vi "Check if config file is valid.vi"(8 "error in (no error)":errorcluster, 10 "Root node":string, 11 "DOM":refnum<k20>) -> (0 "error out":errorcluster)   [LabVIEW 2011, in "COSYLib.lvlib" / "CoSy Config File.lvclass"]
doc: "Checks if a loaded config file appears to be valid (i.e., includes a version number and header information).\nIf the file is invalid, \"error out\" is set to -2628."
uses:
  CoSy Config File.lvclass
  <vilib>/xml/Close Reference(Node).vi
  <vilib>/xml/NI_XML.lvlib
  C:/Program Files (x86)/National Instruments/LabVIEW 2011/resource/objmgr/DOMUserDefRef.rc
  COSYLib.lvlib
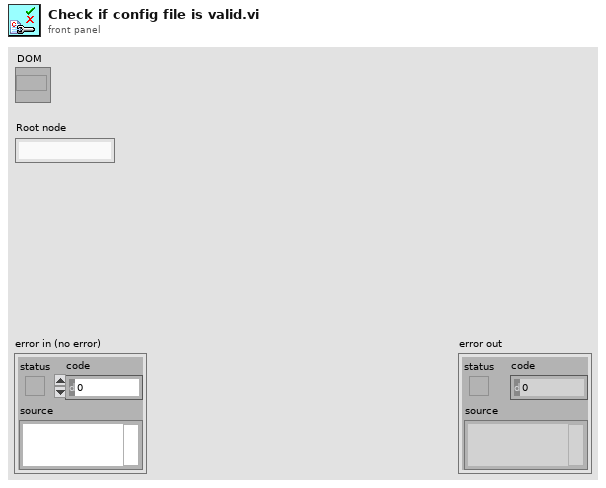
[diagram p1: front panel]
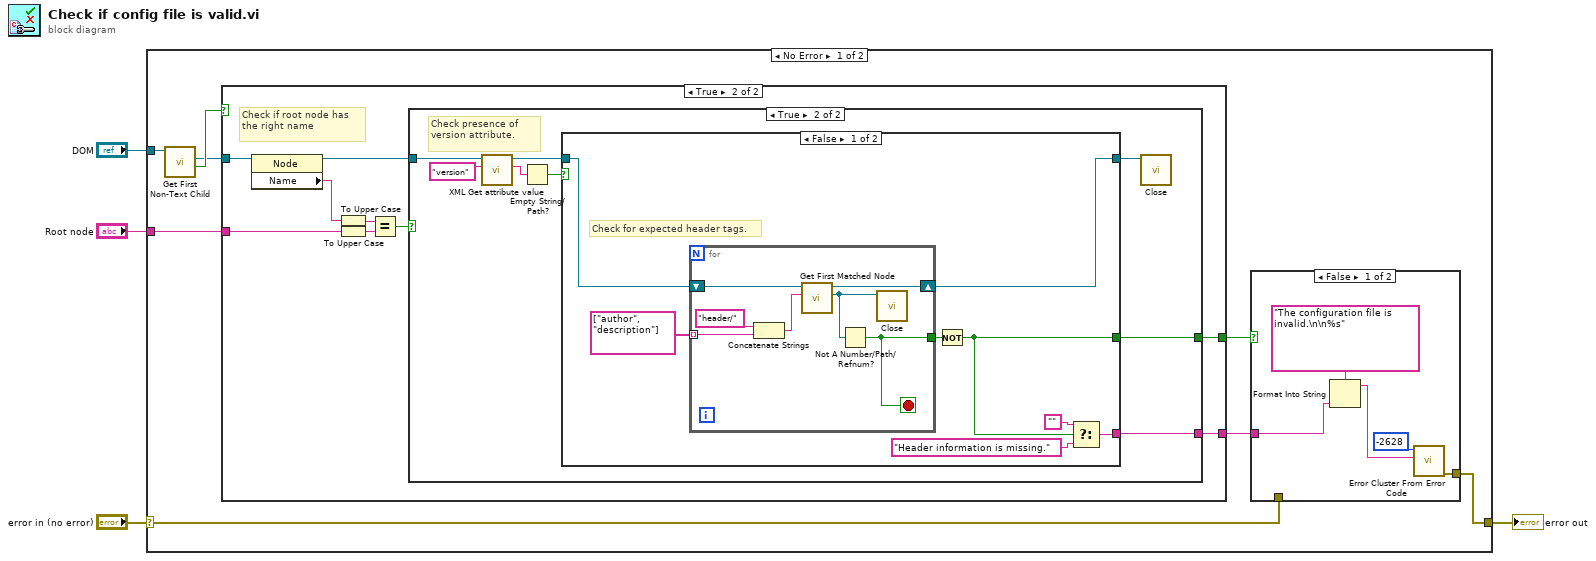
[diagram p0: block diagram]
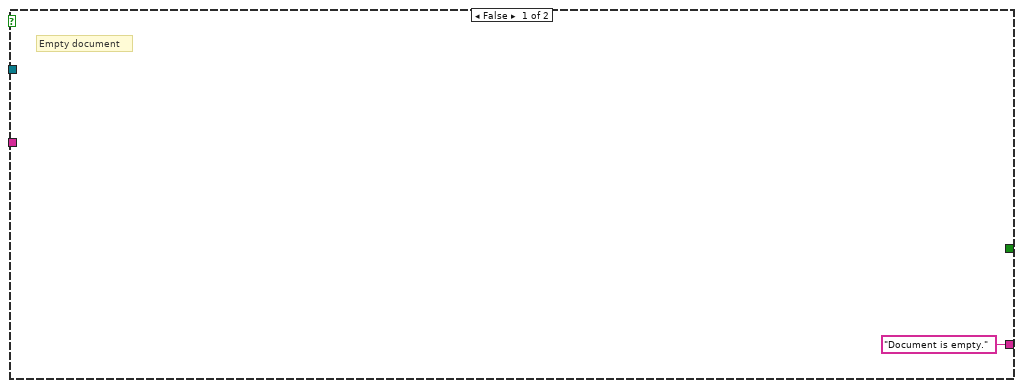
[diagram p3: hidden frame]
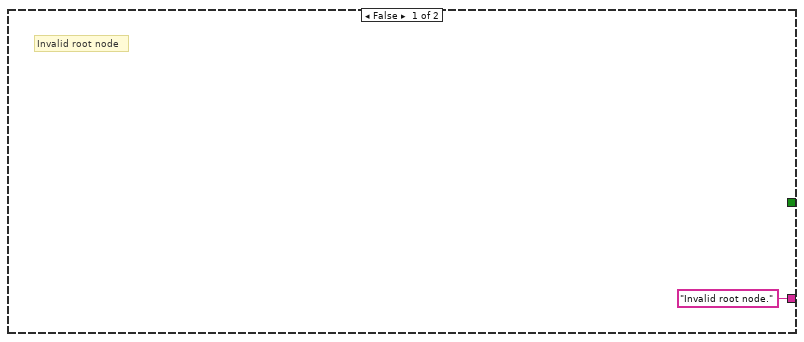
[diagram p4: hidden frame]
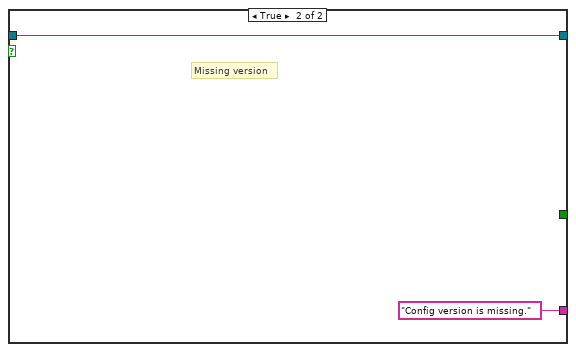
[diagram p5: hidden frame]
diagram:
  n1 = case shown="No Error" "error in (no error)" {
    selector: "error in (no error)" -> [w6 w55]
    tunnel: [w7 w55] -> w3
    tunnel: "DOM" -> [w12 _]
    tunnel: "Root node" -> [w10 _]
    frame No Error {
      n2 = call <vilib>:"Get First Non-Text Child.vi"("node in"=w12) -> ("found child node?"=w11:bool, "child node"=w5:refnum<k20>)  [unwired: 7 in, 2 out]
      n3 = case shown="True" w11 {
        tunnel: w5 -> [_ w28]
        tunnel: w10 -> [_ w27]
        tunnel: [_ w21] -> w9
        tunnel: ["Document is empty." w20] -> w8
        frame False {
          # "Empty document"
        }
        frame True {
          # "Check if root node has the right name"
          n4 = property class="Node"(reference=w28) -> (reference out=w23:refnum<k20>, "Name"=w22:string)  [unwired: 1 in, 1 out]
          n5 = To Upper Case(1:w22) -> (0:w26:string)
          n6 = To Upper Case(1:w27) -> (0:w25:string)
          n7 = Equal?(x=w26, y=w25) -> (x = y?=w24:bool)
          n8 = case shown="True" w24 {
            tunnel: w23 -> [_ w37]
            tunnel: [_ w31] -> w21
            tunnel: ["Invalid root node." w30] -> w20
            frame False {
              # "Invalid root node"
            }
            frame True {
              # "Check presence of version attribute."
              n9 = call "XML Get attribute value.vi"("Attribute name"="version", "Tag node"=w37) -> ("Attribute value"=w35:string, "Tag node out"=w33:refnum<k20>)  [unwired: 7 in, 1 out]
              n10 = Empty String/Path?(string/path=w35) -> (empty?=w34:bool)
              n11 = case shown="False" w34 {
                tunnel: w33 -> [w39 w54]
                tunnel: [w38 w54] -> w32
                tunnel: [w42 _] -> w31
                tunnel: [w44 "Config version is missing."] -> w30
                frame False {
                  # "Check for expected header tags."
                  n12 = for {
                    shift-right: [w51] -> w38
                    shift-left: w39 -> [w52]
                    tunnel: string[] ["author", "description"] -> [w50] mode=indexing
                    tunnel: [w46] -> w43
                    stop <- w46 stop-if-true
                    n13 = Concatenate Strings("header/" ("string"), w50) -> (w49:string)
                    n14 = call <vilib>:"Get First Matched Node.vi"("XPath expression"=w49, "node in"=w52) -> ("node result"=w47:refnum<k20>, "node out"=w51:refnum<k20>)  [unwired: 7 in, 1 out]
                    n15 = Not A Number/Path/Refnum?(number/path/refnum=w47) -> (NaN/Path/Refnum?=w46:bool)
                    n16 = call-poly <vilib>:"Close.vi"("node"=w47) -> ()  [unwired: 8 in, 1 out]
                  }
                  n17 = Not(x=w43) -> (.not. x?=w42:bool)
                  n18 = Select(t="", s=w42, f="Header information is missing.") -> (s? t:f=w44:string)
                }
                frame True {
                  # "Missing version"
                }
              }
              n19 = call-poly <vilib>:"Close.vi"("node"=w32) -> ()  [unwired: 8 in, 1 out]
            }
          }
        }
      }
      n20 = case shown="False" w9 {
        tunnel: w8 -> [w15 _]
        tunnel: [w17 w18] -> w7
        tunnel: w6 -> [_ w18]
        frame False {
          n21 = Format Into String(format string="The configuration file is invalid.\n\n%s", w15) -> (resulting string=w13:string)  [unwired: 2 in, 1 out]
          n22 = call <vilib>:"Error Cluster From Error Code.vi"("error message (\"\")"=w13, "error code (0)"=-2628) -> ("error out"=w17:errorcluster)  [unwired: 7 in]
        }
        frame True {
        }
      }
    }
    frame Error {
    }
  }
  "error out" <- w3
